vi "GetDataEvent_Service.vi"() -> ()   [LabVIEW 2017]
doc: "This is an example of how to read Data Sets from the InsightCM database. Using a similiar method you can read any waveform that has been stored and perform additional analysis on it or save it to a file format."
uses:
  <vilib>/addons/InsightCM/MessageBus/Base/controls/AssetNodeView.ctl
  <vilib>/addons/InsightCM/MessageBus/Base/controls/AssetState.ctl
  <vilib>/addons/InsightCM/MessageBus/Base/controls/Metric.ctl
  <vilib>/addons/InsightCM/MessageBus/Base/controls/KeyValuePair.ctl
  <vilib>/addons/InsightCM/MessageBus/Base/controls/AssetNodeReference.ctl
  <vilib>/addons/InsightCM/MessageBus/Base/controls/DataEvent.ctl
  <vilib>/addons/InsightCM/MessageBus/Base/controls/DataSetByteData.ctl
  <vilib>/addons/InsightCM/MessageBus/Base/controls/TrendPoint.ctl
  <vilib>/addons/InsightCM/MessageBus/MessageService/IcmMessageService.lvclass
panel:
  in  "Seconds from now":i64=3600
  out "error out":errorcluster
  out "Ready?":bool
  out "Asset Name (debug)":string
  out "Command (debug)":string
  out "Output":T2(array[cluster])
  out "TrendPoints":T3[](array[typedef])
  out "DataSets":T4[](array[typedef])
  out "date/time":string
  out "Numeric":i32
  out "DataEvents":T5[](array[typedef])
  out "AssetNodeView":T6
  out "AssetNodes":T6[](array[typedef])
  # "This is an EXE to host a web service for InsightCM.\n\nUsage:  http://127.0.0.1:8002/Query/GetLastEvent?Asset=<AssetName>\n\nOutput: Last event for the asset within X days, all channels (JSON)"
  # "1 hr = 3600, 1 day = 86400"
  # "This example shows how to query InsightCM data.\n\n1) Click Refresh to load assets.\n2) Select an asset.\n3) Select a data event and a sensor.\n\nNote: If the sensor does not have waveform data, the waveform graph will be empty."
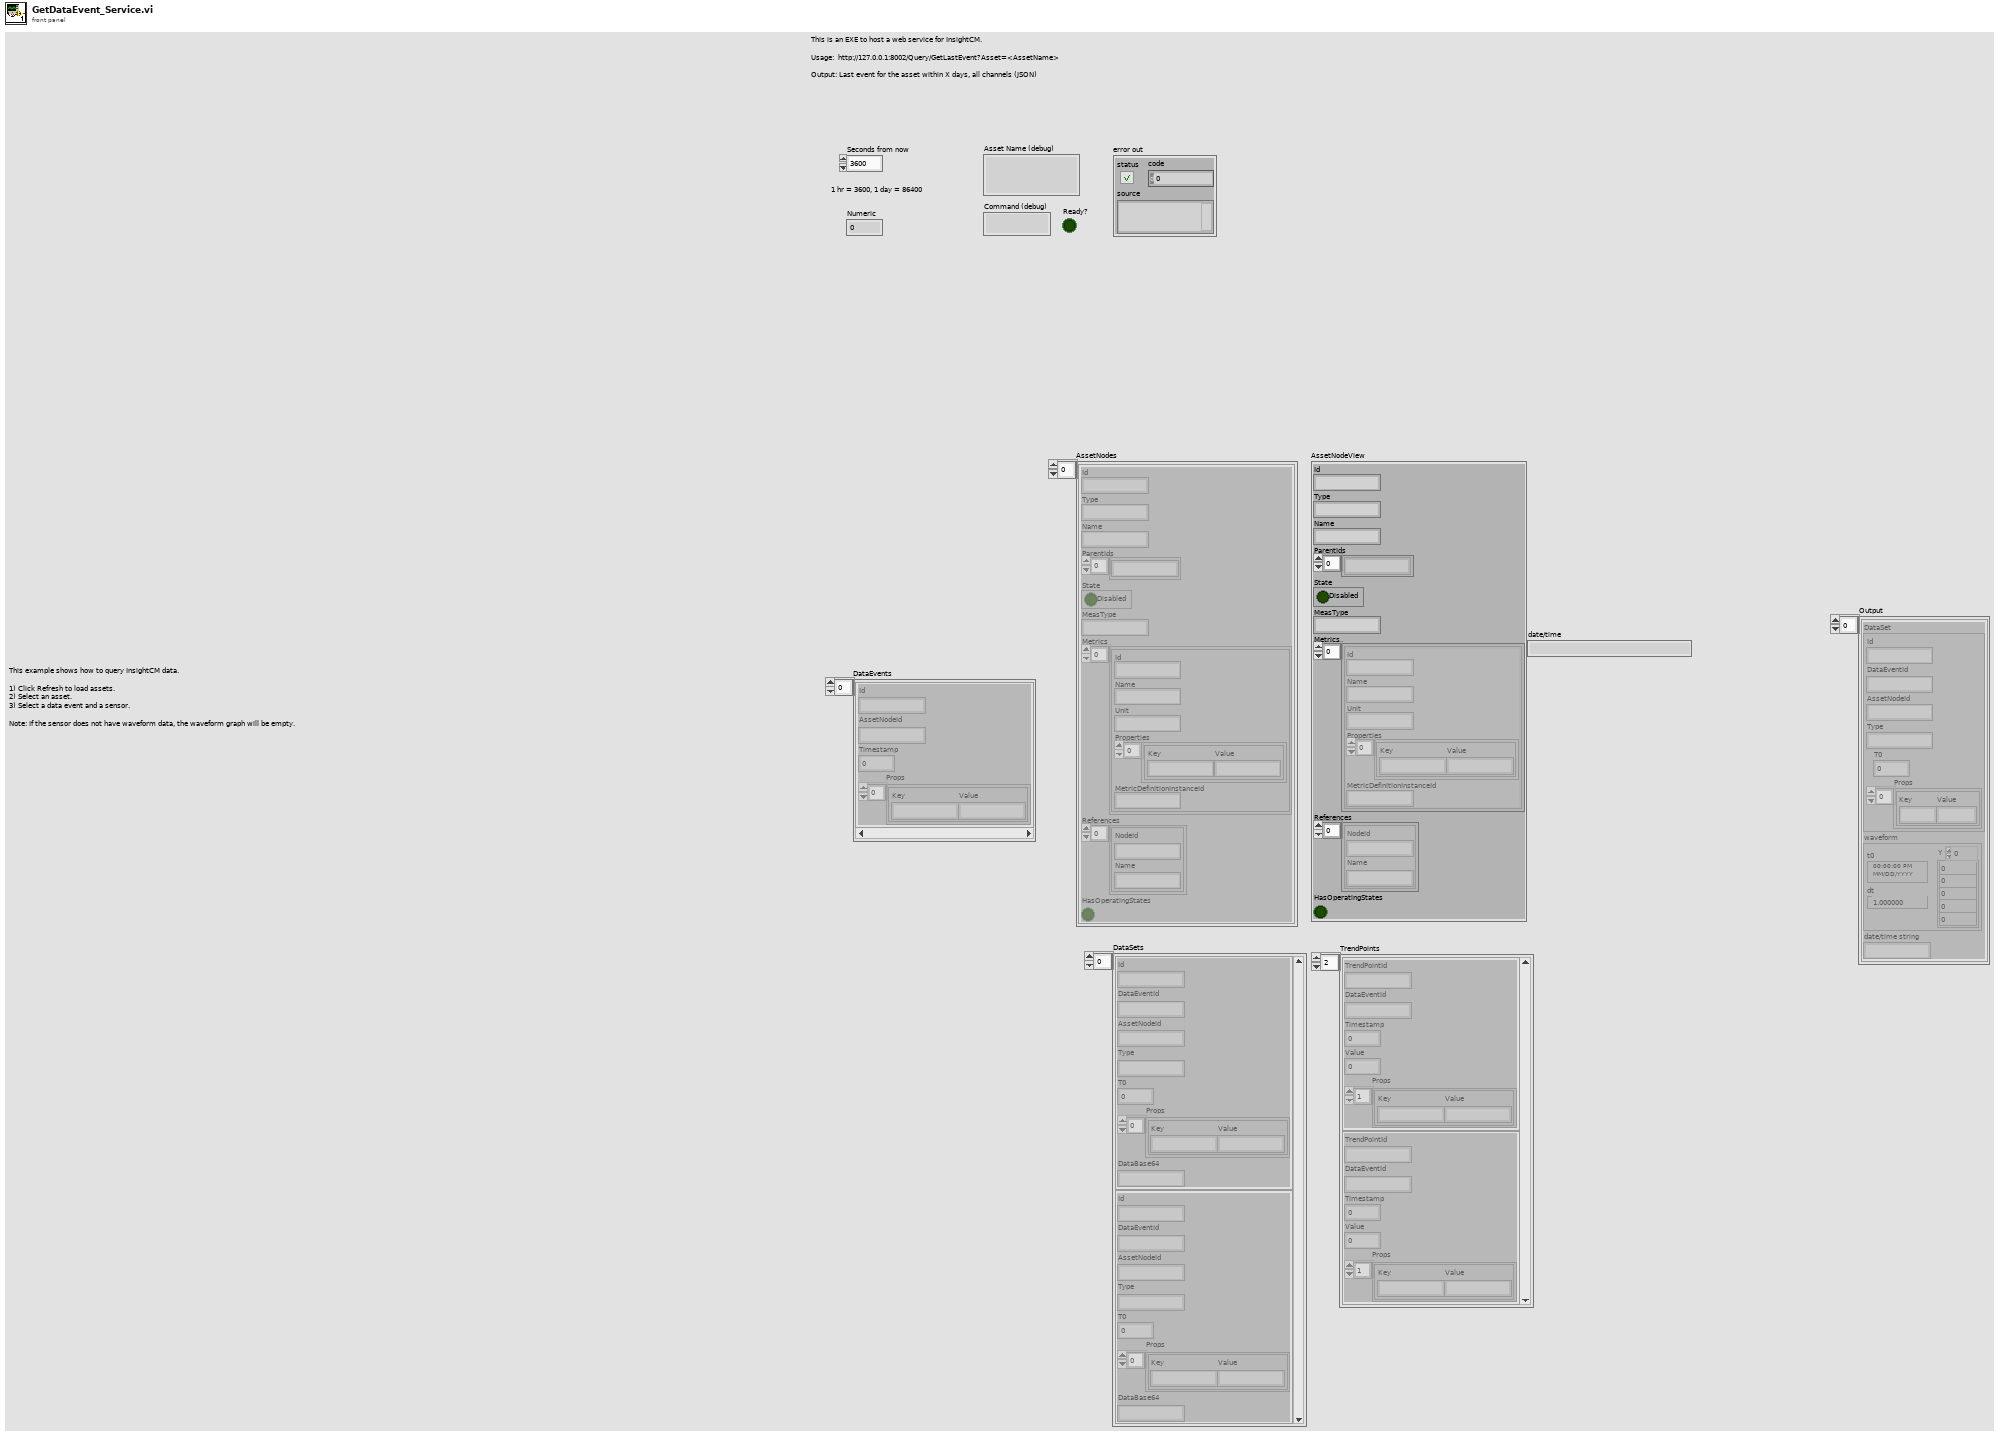
[diagram p1: front panel]
types:
  T1 = typedef "KeyValuePair.ctl" = cluster{"Key":string, "Value":string}
  T2 = cluster{"DataSet":cluster{"Id":string, "DataEventId":string, "AssetNodeId":string, "Type":string, "T0":i64, "Props":T1[]}, "waveform":waveform(sgl), "date/time string":string}[]
  T3 = typedef "TrendPoint.ctl" = cluster{"TrendPointId":string, "DataEventId":string, "Timestamp":i64, "Value":dbl, "Props":T1[]}
  T4 = typedef "DataSetByteData.ctl" = cluster{"Id":string, "DataEventId":string, "AssetNodeId":string, "Type":string, "T0":i64, "Props":T1[], "DataBase64":string}
  T5 = typedef "DataEvent.ctl" = cluster{"Id":string, "AssetNodeId":string, "Timestamp":i64, "Props":T1[]}
  T6 = typedef "AssetNodeView.ctl" = cluster{"Id":string, "Type":string, "Name":string, "ParentIds":string[], "State":T7, "MeasType":string, "Metrics":T8[], "References":T9[], "HasOperatingStates":bool}
  T7 = typedef "AssetState.ctl" = cluster{"Disabled":bool}
  T8 = typedef "Metric.ctl" = cluster{"Id":string, "Name":string, "Unit":string, "Properties":T1[], "MetricDefinitionInstanceId":string}
  T9 = typedef "AssetNodeReference.ctl" = cluster{"NodeId":string, "Name":string}
  T10 = cluster{"Id":string, "DataEventId":string, "AssetNodeId":string, "Type":string, "T0":i64, "Props":T1[]}
  T11 = cluster{"DataSet":cluster{"Id":string, "DataEventId":string, "AssetNodeId":string, "Type":string, "T0":i64, "Props":T1[]}, "waveform":waveform(sgl), "date/time string":string}
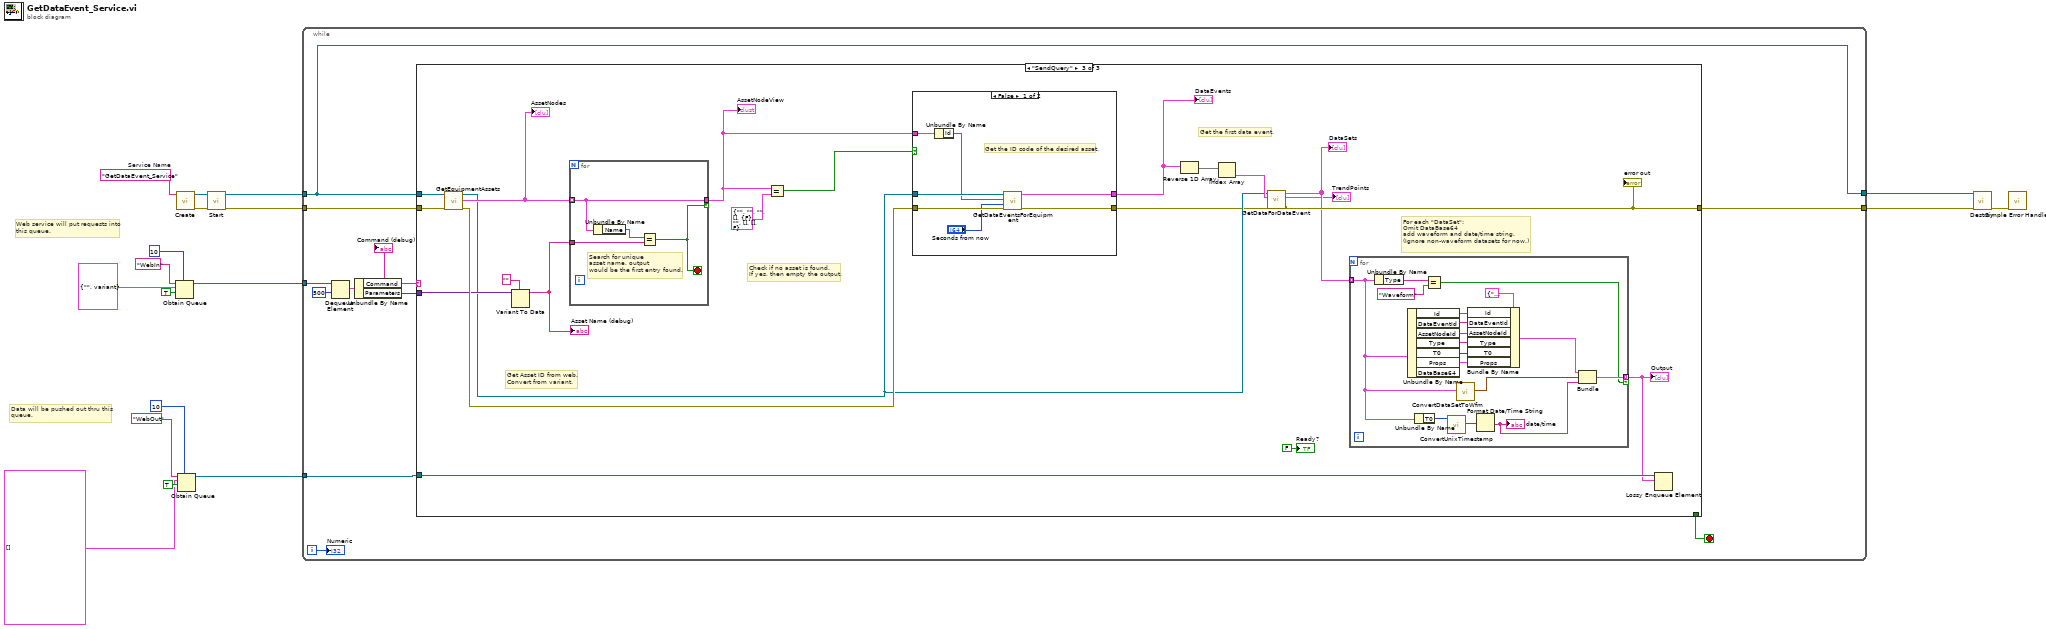
[diagram p0: block diagram]
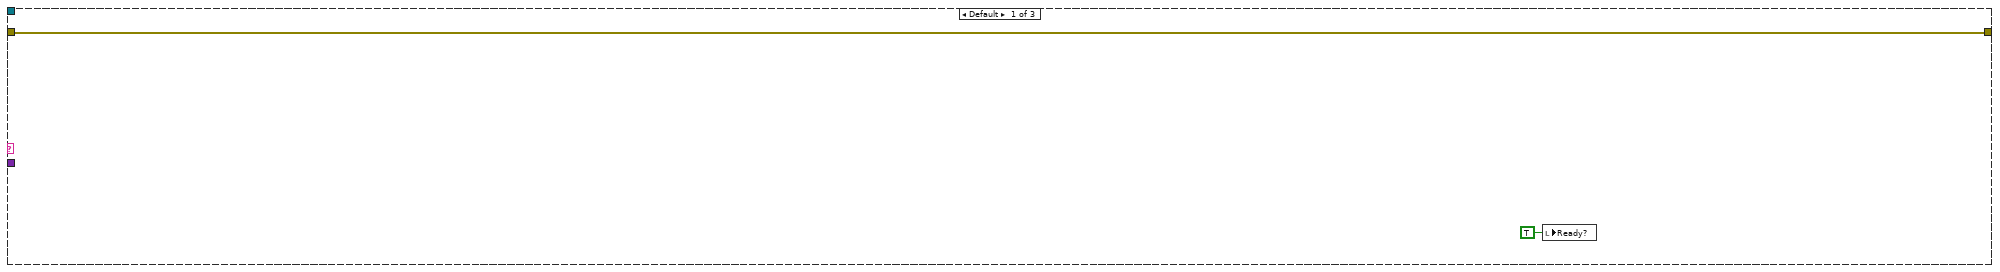
[diagram p2: hidden frame]
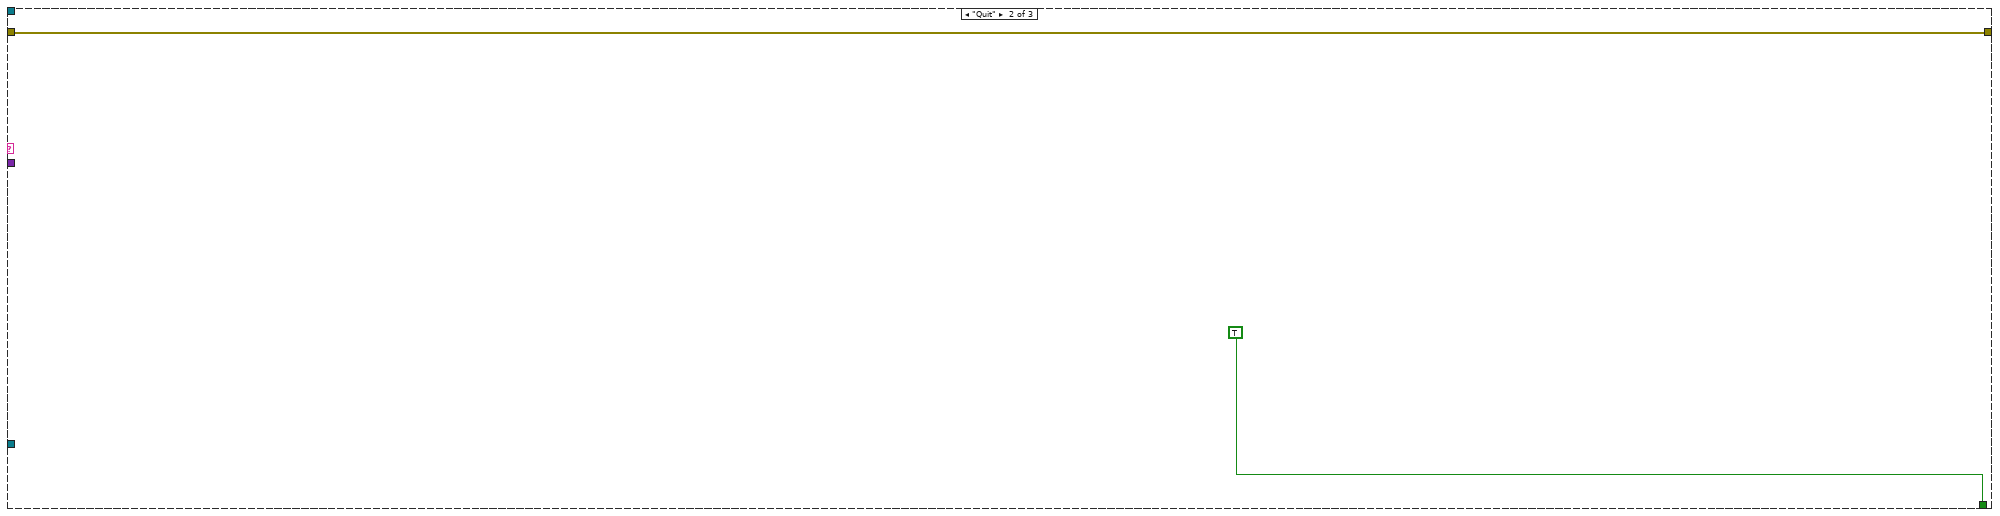
[diagram p3: hidden frame]
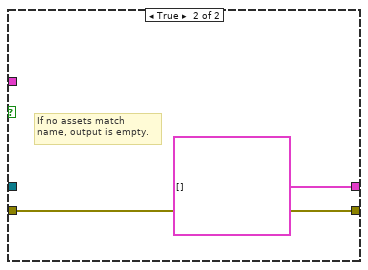
[diagram p4: hidden frame]
diagram:
  w18 = "GetDataEvent_Service"  # Service Name
  # "Data will be pushed out thru this\nqueue."
  # "Web service will put requests into\nthis queue."
  n1 = Obtain Queue(max queue size (-1, unlimited)=10, name (unnamed)="WebIn", element data type=cluster{"Command":string, "Parameters":variant} {"Command"="", "Parameters"=variant}, create if not found? (T)=TRUE) -> (queue out=w8:refnum<queue>)  [unwired: 1 in, 2 out]
  n2 = call <vilib>:"Create.vi"("service name"=w18) -> ("error out"=w13:errorcluster, "service out"=w14:refnum<class "IcmMessageService.lvclass">)  [unwired: 9 in]
  n3 = Obtain Queue(max queue size (-1, unlimited)=10, name (unnamed)="WebOut", element data type=T2 [] ("Output"), create if not found? (T)=TRUE) -> (queue out=w7:refnum<queue>)  [unwired: 1 in, 2 out]
  n4 = call <vilib>:"Start.vi"("error in (no error)"=w13, "service in"=w14) -> ("error out"=w11:errorcluster, "service out"=w12:refnum<class "IcmMessageService.lvclass">)  [unwired: 8 in]
  n5 = while {
    tunnel: w12 -> [w28]
    tunnel: w11 -> [w29]
    tunnel: [w28] -> w15
    tunnel: [w27] -> w16
    tunnel: w8 -> [w26]
    tunnel: w7 -> [w24]
    i -> [w19]
    stop <- w23 stop-if-true
    n6 = Dequeue Element(queue=w26, timeout in ms (-1)=500) -> (element=w22:cluster{"Command":string, "Parameters":variant})  [unwired: 1 in, 3 out]
    n7 = Unbundle By Name(w22) -> ("Command"=w21:string, "Parameters"=w20:variant)
    "Command (debug)" <- w21
    n8 = case shown="\"SendQuery\"" w21 {
      tunnel: w29 -> [w31 w33 w53]
      tunnel: w28 -> [_ _ w40]
      tunnel: [w31 w33 w38] -> w27
      tunnel: w24 -> [_ _ w47]
      tunnel: [_ TRUE _] -> w23
      tunnel: w20 -> [_ _ w46]
      frame Default {
        n9 = local write "Ready?"(TRUE ("Ready?")) -> ()
      }
      frame "Quit" {
      }
      frame "SendQuery" {
        # "For each \"DataSet\":\nOmit DataBase64\nadd waveform and date/time string.\n(Ignore non-waveform datasets for now.)"
        # "Get Asset ID from web.\nConvert from variant."
        # "Get the first data event."
        # "Check if no asset is found.\nIf yes, then empty the output."
        n10 = call "GetEquipmentAssets.vi"("error in (no error)"=w53, "service"=w40) -> ("error out"=w49:errorcluster, "AssetNodes"=w52:T6[])  [unwired: 8 in]
        "AssetNodes" <- w52
        n11 = Variant To Data(type="", Variant=w46) -> (data=w44:string)  [unwired: 1 in, 1 out]
        "Asset Name (debug)" <- w44
        n12 = for {
          tunnel: w52 -> [w81] mode=indexing
          tunnel: w44 -> [w82]
          tunnel: [w81] -> w50 if=w80
          stop <- w80 stop-if-true
          # "Search for unique \nasset name, output\nwould be the first entry found."
          n13 = Unbundle By Name(w81) -> ("Name"=w83:string)
          n14 = Equal?(x=w83, y=w82) -> (x = y?=w80:bool)
        }
        "AssetNodeView" <- w50
        n15 = Equal?(x=w50, y=T6 {"Id"="", "Type"="", "Name"="", "ParentIds"=[], "State"={"Disabled"=FALSE}, "MeasType"="", "Metrics"=[], "References"=[], "HasOperatingStates"=FALSE} ("AssetNodeView 2")) -> (x = y?=w48:bool)
        n16 = case shown="False" w48 {
          tunnel: w50 -> [w75 _]
          tunnel: w40 -> [w77 _]
          tunnel: w49 -> [w76 w78]
          tunnel: [w74 T5[] [] ("DataEvents")] -> w43
          tunnel: [w73 w78] -> w39
          frame False {
            # "Get the ID code of the desired asset."
            n17 = Unbundle By Name(w75) -> ("Id"=w72:string)
            n18 = call "GetDataEventsForEquipment.vi"("error in (no error)"=w76, "sec per day"="Seconds from now", "equipment id"=w72, "service"=w77) -> ("error out"=w73:errorcluster, "DataEvents"=w74:T5[])  [unwired: 6 in]
          }
          frame True {
            # "If no assets match\nname, output is empty."
          }
        }
        "DataEvents" <- w43
        n19 = Reverse 1D Array(array=w43) -> (reversed array=w42:T5[])
        n20 = Index Array(array=w42) -> (element=w41:T5)  [unwired: 1 in]
        n21 = call "GetDataForDataEvent.vi"("error in (no error)"=w39, "DataEvent"=w41, "service"=w40) -> ("error out"=w38:errorcluster, "TrendPoints"=→"TrendPoints":T3[], "DataSets"=w37:T4[])  [unwired: 6 in]
        "DataSets" <- w37
        "error out" <- w38
        n22 = for {
          tunnel: w37 -> [w62] mode=indexing
          tunnel: [w64] -> w35 mode=indexing if=w63
          n23 = Unbundle By Name(w62) -> ("Type"=w70:string)
          n24 = Unbundle By Name(w62) -> ("Id"=w60:string, "DataEventId"=w56:string, "AssetNodeId"=w57:string, "Type"=w58:string, "T0"=w59:i64, "Props"=w55:T1[])  [unwired: 1 out]
          n25 = Unbundle By Name(w62) -> ("T0"=w68:i64)
          n26 = Equal?(x=w70, y="Waveform") -> (x = y?=w63:bool)
          n27 = call <vilib>:"ConvertUnixTimestamp.vi"("Timestamp in"=w68) -> ("Time Stamp out"=w67:timestamp)  [unwired: 10 in]
          n28 = call "ConvertDataSetToWfm.vi"("DataSet"=w62) -> ("waveform"=w66:waveform(sgl))  [unwired: 10 in]
          n29 = Bundle By Name(cluster=T10 {"Id"="", "DataEventId"="", "AssetNodeId"="", "Type"="", "T0"=0, "Props"=[]} ("DataSet"), "Id"=w60, "DataEventId"=w56, "AssetNodeId"=w57, "Type"=w58, "T0"=w59, "Props"=w55) -> (w54:T10)
          n30 = Format Date/Time String(seconds (now)=w67) -> (date/time string=w65:string)  [unwired: 2 in]
          "date/time" <- w65
          n31 = Bundle("DataSet"=w54, "waveform"=w66, "date/time string"=w65) -> (w64:T11)  [unwired: 1 in]
        }
        "Output" <- w35
        n32 = Lossy Enqueue Element(queue=w47, element=w35) -> ()  [unwired: 1 in, 4 out]
        "Ready?" <- FALSE ("Ready?")
      }
    }
    "Numeric" <- w19
  }
  n33 = call <vilib>:"Destroy.vi"("error in (no error)"=w16, "service in"=w15) -> ("error out"=w17:errorcluster)  [unwired: 9 in]
  n34 = call <vilib>:"Simple Error Handler.vi"("error in (no error)"=w17) -> ()  [unwired: 4 in, 5 out]
